vi "Main.vi"() -> ()   [LabVIEW 2015]
doc: "The myRIO Project template acquires acceleration data from the onboard accelerometer and displays the changes of acceleration values in a waveform chart."
uses:
  <vilib>/myRIO/Instrument Drivers/Onboard IO/PWM/typedefs/PWM Reference.ctl
  <vilib>/myRIO/Common/Instrument Driver Framework/Utilities/typedefs/myRIO Generic Hardware Reference.ctl
  <vilib>/myRIO/Common/Instrument Driver Framework/Utilities/typedefs/Hardware Version Enum.ctl
  <vilib>/myRIO/Common/Instrument Driver Framework/Utilities/typedefs/myRIO v1.0 Reference.ctl
  <vilib>/myRIO/Common/Instrument Driver Framework/Utilities/typedefs/Generic FPGA Reference.ctl
  <vilib>/myRIO/Common/Instrument Driver Framework/myRIO v1.0/PWM/typedefs/PWM Channels Enum.ctl
  <vilib>/myRIO/Instrument Drivers/Onboard IO/PWM/typedefs/PWM Configuration.ctl
  <vilib>/userdefined/High Color/nirio_resource_hc.ctl
  <vilib>/myRIO/Common/Instrument Driver Framework/Utilities/vis/Is FPGA Ref Available.vi
  <vilib>/myRIO/Common/Instrument Driver Framework/myRIO v1.0/PWM/vis/myRIO v1.1 Open PWM.vi
  <vilib>/myRIO/Instrument Drivers/Onboard IO/PWM/vis/Set Duty Cycle and Frequency.vi
  <vilib>/myRIO/Common/Instrument Driver Framework/Utilities/vis/Validate Channels.vi
  <vilib>/myRIO/Common/Instrument Driver Framework/myRIO v1.0/PWM/vis/myRIO v1.0 Reserve PWM.vi
  <vilib>/myRIO/Common/Instrument Driver Framework/myRIO v1.0/UART/vis/myRIO v1.0 Close UART.vi
  <vilib>/myRIO/Common/Instrument Driver Framework/myRIO v1.0/PWM/vis/myRIO v1.0 Build MUX Configuration PWM.vi
  <vilib>/myRIO/Common/Instrument Driver Framework/myRIO v1.0/Resource Manager/vis/myRIO v1.0 Reserve Channel List.vi
  <vilib>/myRIO/Common/Instrument Driver Framework/myRIO v1.0/Resource Manager/vis/myRIO v1.0 Create Configuration List.vi
  <vilib>/myRIO/Common/Instrument Driver Framework/myRIO v1.0/Resource Manager/vis/myRIO v1.0 Reserve Channel.vi
  <vilib>/myRIO/Common/Instrument Driver Framework/myRIO v1.0/Resource Manager/vis/myRIO v1.0 Unreserve Channel.vi
  <vilib>/myRIO/Common/Instrument Driver Framework/myRIO v1.0/Resource Manager/vis/myRIO v1.0 Build Mutex Name.vi
  <vilib>/Utility/VariantDataType/GetNumericInfo.vi
  <vilib>/Utility/error.llb/Error Cluster From Error Code.vi
  <vilib>/myRIO/Common/Instrument Driver Framework/myRIO v1.0/myRIO v1.1 Open.vi
  <vilib>/myRIO/Common/Instrument Driver Framework/Utilities/vis/IO Manager.vi
  <vilib>/myRIO/Common/Instrument Driver Framework/Utilities/vis/Configuration Manager.vi
  <vilib>/myRIO/Common/Instrument Driver Framework/myRIO v1.0/Resource Manager/vis/myRIO v1.0 Configure IO.vi
  <vilib>/myRIO/Common/Instrument Driver Framework/myRIO v1.0/myRIO v1.0 Close.vi
  <vilib>/myRIO/Common/Instrument Driver Framework/myRIO v1.0/PWM/vis/myRIO v1.0 Write PWM.vi
  <vilib>/myRIO/Common/Instrument Driver Framework/Utilities/vis/FPGA Ref Manager.vi
  <vilib>/myRIO/Common/Instrument Driver Framework/myRIO v1.0/myRIO v1.0 Reset FPGA.vi
  <vilib>/myRIO/Common/Instrument Driver Framework/myRIO v1.0/IRQ/vis/myRIO v1.0 IRQ Info FGV.vi
  <vilib>/myRIO/Common/Instrument Driver Framework/myRIO v1.0/IRQ/vis/myRIO v1.0 Timer IRQ Info FGV.vi
  <vilib>/myRIO/Common/Instrument Driver Framework/myRIO v1.0/IRQ/vis/myRIO v1.0 ISR Agent.vi
  <vilib>/myRIO/Express VI/Onboard IO/PWM/PWM Express VI.xnode
  <vilib>/myRIO/Instrument Drivers/Onboard IO/PWM/vis/myRIO PWM Open.xnode
  <vilib>/myRIO/Instrument Drivers/Utilities/Utilities.lvlib
  <vilib>/myRIO/Instrument Drivers/Onboard IO/PWM/PWM.lvlib
panel:
  out "Numeric Control 3":i32
  out "error out 5":errorcluster
  out "error out 4":errorcluster
  out "compass 2":dbl format="%#_13g"
  in  "error in (no error) 2":errorcluster
  in  "Duty Cycle 2":dbl=0.5
  in  "error in (no error)":errorcluster
  in  "Duty Cycle":dbl=0.5
  out "compass 1":dbl format="%#_13g"
  out "error out":errorcluster
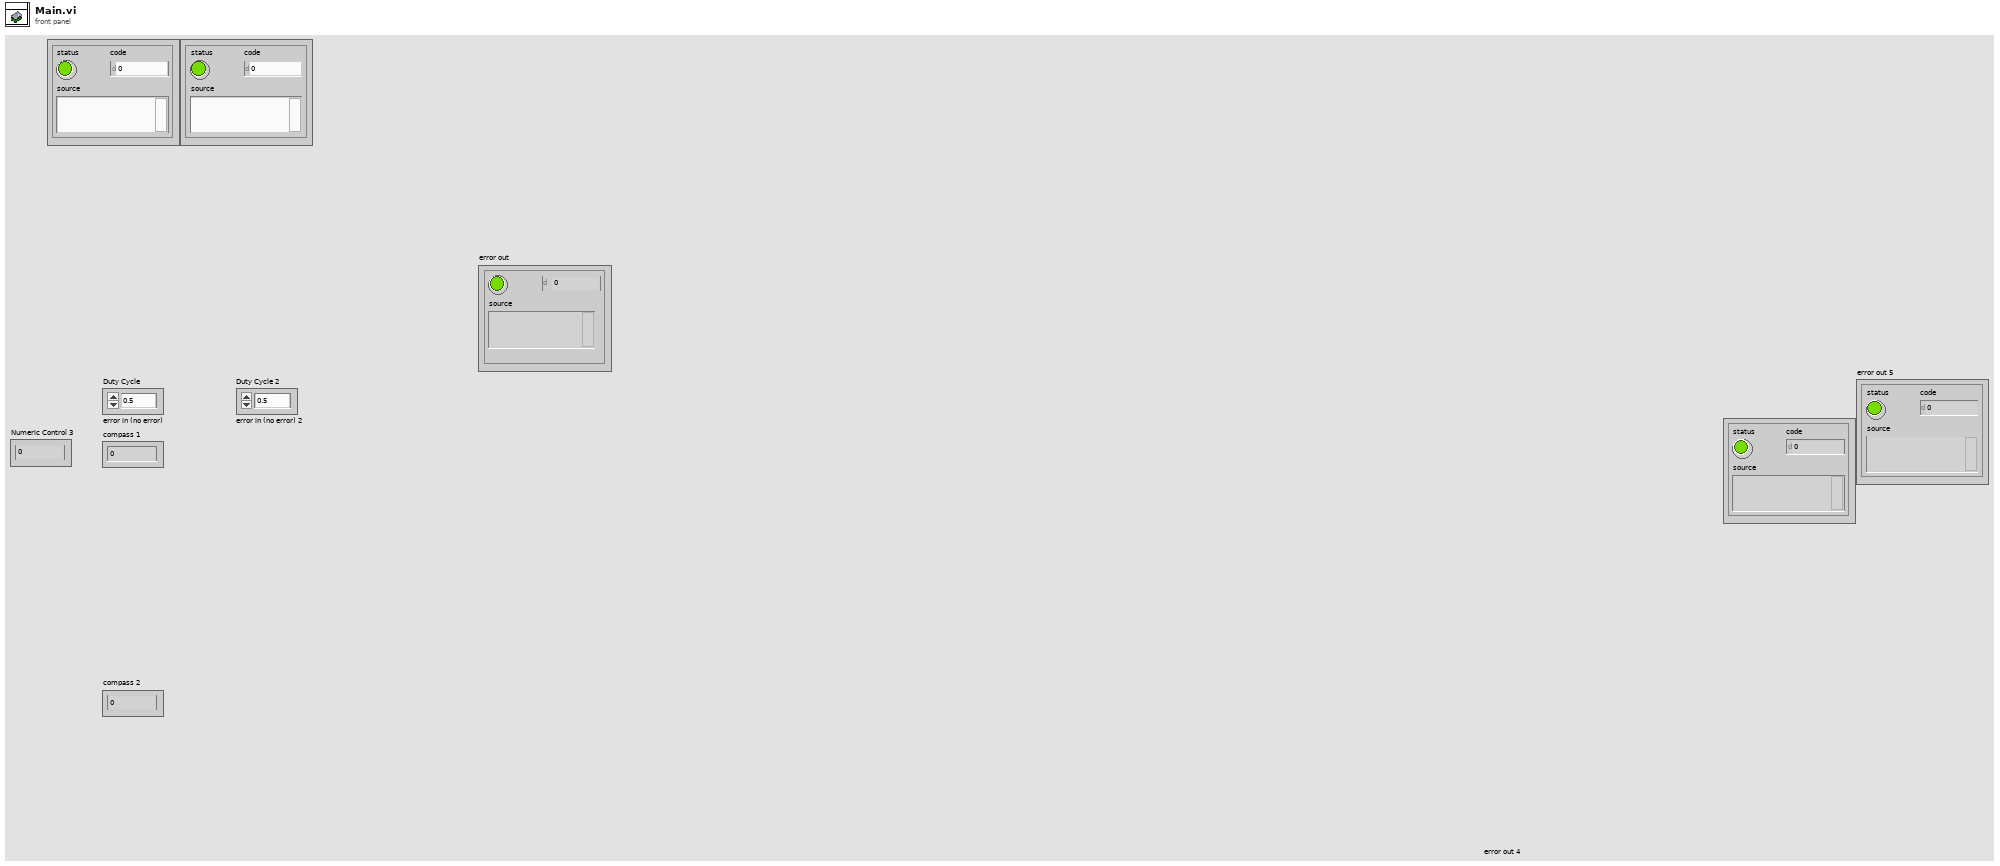
[diagram p1: front panel]
types:
  T1 = typedef "PWM.lvlib/PWM Reference.ctl" = cluster{"myRIO Reference":T2, "PWM Channels Enum":T6, "PWM Configuration":T7}
  T2 = typedef "myRIO Generic Hardware Reference.ctl" = cluster{"myRIO Model":T3, "myRIO Hardware Reference":T4}
  T3 = typedef "Hardware Version Enum.ctl" = enum16{"Unknown", "myRIO-1900", "myRIO-1950", "roboRIO"}
  T4 = typedef "myRIO v1.0 Reference.ctl" = cluster{"Generic FPGA Reference":T5, "Allow multiple opens":bool}
  T5 = typedef "Generic FPGA Reference.ctl" = refnum<k20>
  T6 = typedef "PWM Channels Enum.ctl" = enum16{"Not Connected", "C/PWM0", "C/PWM1", "A/PWM0", "A/PWM1", "A/PWM2", "B/PWM0", "B/PWM1", "B/PWM2", "PWM/PWM0", "PWM/PWM1", "PWM/PWM2", "PWM/PWM3", "PWM/PWM4", "PWM/PWM5", "PWM/PWM6", "PWM/PWM7", "PWM/PWM8", "PWM/PWM9"}
  T7 = typedef "PWM.lvlib/PWM Configuration.ctl" = cluster{"Frequency":dbl, "Duty Cycle":dbl}
  T8 = typedef "nirio_resource_hc.ctl" = tag
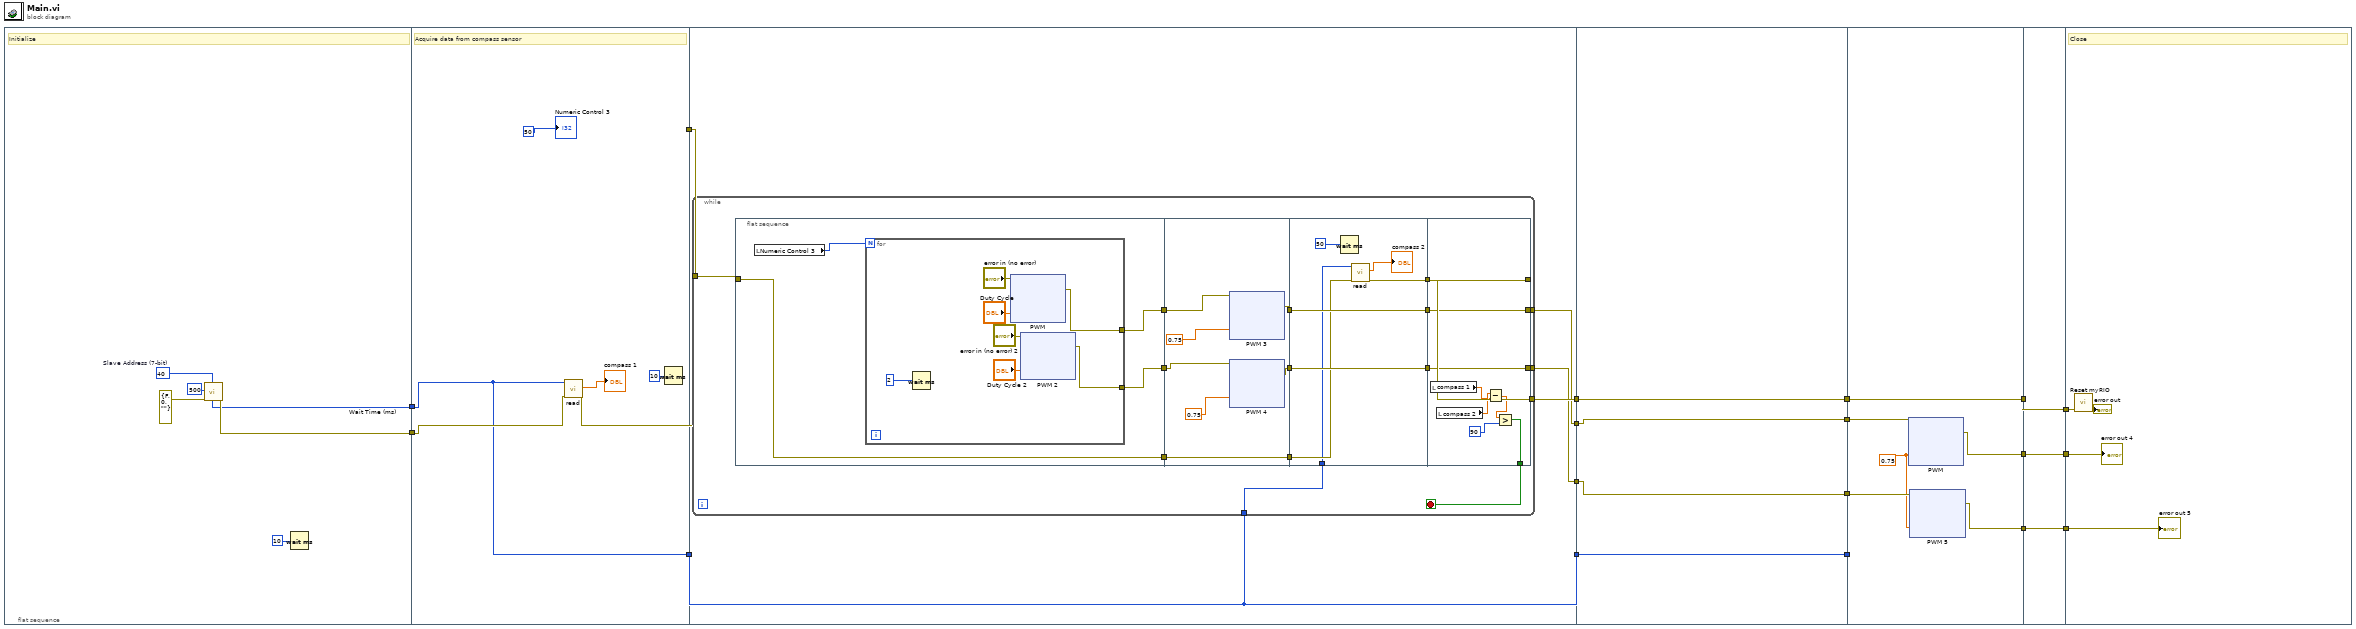
[diagram p0: block diagram]
diagram:
  n1 = flat-sequence {
    tunnel: [w20] -> w18
    tunnel: [w21] -> w17
    tunnel: w18 -> [w25]
    tunnel: w17 -> [w27]
    tunnel: [w26] -> w16
    tunnel: [w25] -> w15
    tunnel: [w32] -> w14
    tunnel: w16 -> [w34]
    tunnel: w15 -> [w33]
    tunnel: [w33] -> w13
    tunnel: [w31] -> w12
    tunnel: [w30] -> w11
    tunnel: w14 -> [w226]
    tunnel: [w226] -> w10
    tunnel: w13 -> [w225]
    tunnel: [w225] -> w9
    tunnel: w12 -> [w224]
    tunnel: w11 -> [w223]
    tunnel: [w224] -> w6
    tunnel: [w223] -> w5
    tunnel: w10 -> [w232]
    tunnel: w9 -> [_]
    tunnel: [w232] -> w8
    tunnel: w6 -> [w231]
    tunnel: w5 -> [w230]
    tunnel: [w229] -> w3
    tunnel: [w228] -> w1
    tunnel: [w305] -> w7
    tunnel: w8 -> [w305]
    tunnel: [w304] -> w4
    tunnel: w3 -> [w304]
    tunnel: [w303] -> w2
    tunnel: w1 -> [w303]
    tunnel: w7 -> [w308]
    tunnel: w4 -> [w307]
    tunnel: w2 -> [w306]
    frame #0 {
      w20 = u8 40  # Slave Address (7-bit)
      # "Initialize"
      n2 = call "Wait Time (ms).vi"("error in (no error)"=errorcluster {"status"=FALSE, "code"=0, "source"=""} ("error in"), "Wait Time (ms)"=u32 500) -> ("error out"=w21:errorcluster)  [unwired: 9 in]
      n3 = Wait (ms)(milliseconds to wait=10) -> ()  [unwired: 1 out]
    }
    frame #1 {
      # "Acquire data from compass sensor"
      n4 = call "read.vi"("error in (no error)"=w27, "Slave Address (7-bit)"=w25) -> ("error out"=w26:errorcluster, "Numeric"=→"compass 1":dbl)  [unwired: 7 in, 1 out]
      n5 = Wait (ms)(milliseconds to wait=u32 10) -> ()  [unwired: 1 out]
      "Numeric Control 3" <- 50
    }
    frame #2 {
      n6 = while {
        tunnel: w34 -> [w49]
        tunnel: w33 -> [w48]
        tunnel: [w43] -> w32
        tunnel: [w42] -> w31
        tunnel: [w41] -> w30
        stop <- w44 stop-if-true
        n7 = flat-sequence {
          tunnel: [w53] -> w40
          tunnel: [w52] -> w38
          tunnel: [w51] -> w36
          tunnel: w49 -> [w51]
          tunnel: w40 -> [w134]
          tunnel: [w131] -> w39
          tunnel: w38 -> [w133]
          tunnel: [w132] -> w37
          tunnel: w36 -> [w137]
          tunnel: [w137] -> w35
          tunnel: w39 -> [w214]
          tunnel: w37 -> [w213]
          tunnel: w35 -> [w212]
          tunnel: w48 -> [w209]
          tunnel: [w214] -> w47
          tunnel: [w213] -> w46
          tunnel: [w211] -> w45
          tunnel: [w220] -> w43
          tunnel: [w221] -> w41
          tunnel: [w222] -> w42
          tunnel: w47 -> [w222]
          tunnel: w46 -> [w221]
          tunnel: w45 -> [w220]
          tunnel: [w215] -> w44
          frame #0 {
            n8 = local read "Numeric Control 3"() -> (w50:i32)
            n9 = for {
              N: w50 -> [_]
              tunnel: [w60] -> w53
              tunnel: [w59] -> w52
              n10 = Wait (ms)(milliseconds to wait=2) -> ()  [unwired: 1 out]
              n11 = xnode "PWM"("Duty Cycle"="Duty Cycle", "error in (no error)"="error in (no error)") -> ("error out"=w60:errorcluster)
              n12 = xnode "PWM 2"("Duty Cycle"="Duty Cycle 2", "error in (no error)"="error in (no error) 2") -> ("error out"=w59:errorcluster)
            }
          }
          frame #1 {
            n13 = xnode "PWM 3"("Duty Cycle"=0.75 ("Duty Cycle 3"), "error in (no error)"=w134) -> ("error out"=w131:errorcluster)
            n14 = xnode "PWM 4"("Duty Cycle"=0.75 ("Duty Cycle 4"), "error in (no error)"=w133) -> ("error out"=w132:errorcluster)
          }
          frame #2 {
            n15 = Wait (ms)(milliseconds to wait=50) -> ()  [unwired: 1 out]
            n16 = call "read.vi"("error in (no error)"=w212, "Slave Address (7-bit)"=w209) -> ("error out"=w211:errorcluster, "Numeric"=→"compass 2":dbl)  [unwired: 7 in, 1 out]
          }
          frame #3 {
            n17 = local read "compass 1"() -> (w218:dbl)
            n18 = local read "compass 2"() -> (w219:dbl)
            n19 = Subtract(x=w219, y=w218) -> (x-y=w217:dbl)
            n20 = Greater?(x=w217, y=90) -> (0:w215:bool)
          }
        }
      }
    }
    frame #3 {
    }
    frame #4 {
      w227 = 0.75
      n21 = xnode "PWM"("Duty Cycle"=w227, "error in (no error)"=w231) -> ("error out"=w229:errorcluster)
      n22 = xnode "PWM 5"("Duty Cycle"=w227, "error in (no error)"=w230) -> ("error out"=w228:errorcluster)
    }
    frame #5 {
    }
    frame #6 {
      # "Close"
      n23 = call <vilib>:"Reset myRIO.vi"("error in (no error)"=w308) -> ("error out"=→"error out":errorcluster)  [unwired: 10 in]
      "error out 4" <- w307
      "error out 5" <- w306
    }
  }
